vi "QueryMarker.vi"(8 "error in (no error)":errorcluster, 11 "Keysight44xx in":refnum<class "Keysight44xx.lvclass">) -> (0 "error out":errorcluster, 1 "MarkerPosition":dbl, 2 "MarkerAmplitude":dbl, 3 "Keysight44xx out":refnum<class "Keysight44xx.lvclass">)   [LabVIEW 2018, in "SpecAnPlugins.lvlib" / "Keysight44xx.lvclass"]
uses:
  Keysight44xx.lvclass
  C:/Users/ico/Documents/Projects/NistPluggableModules/SpecAn/SpecAnPlugins/SpecAnBaseClass/SpecAnBase.lvclass
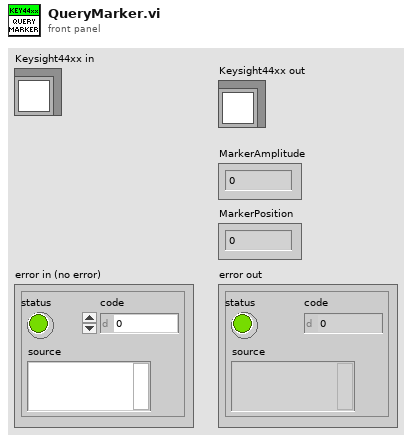
[diagram p1: front panel]
types:
  T1 = typedef "SpecAnPlugins.lvlib/SpecAnBase.lvclass/Acquisition.ctl" = cluster{"Handle":string, "Connected":bool, "Enabled":bool, "SweepModeContinuous":bool, "NumberOfSweeps":i32, "DetectorTypeAuto":bool, "DetectorType":i32, "VerticalScale":i32, "MaximumTime(seconds)":dbl}
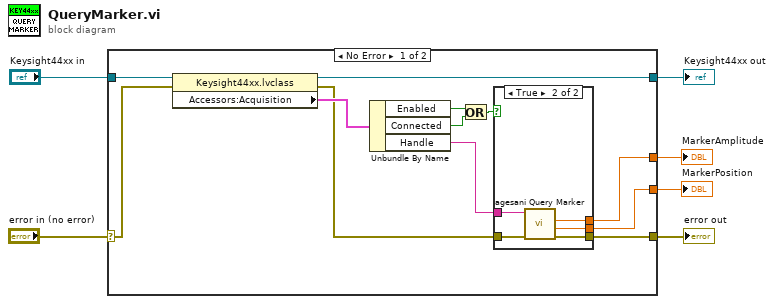
[diagram p0: block diagram]
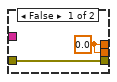
[diagram p2: hidden frame]
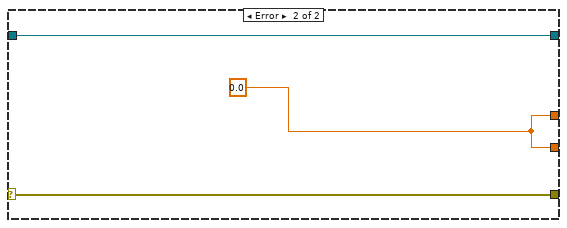
[diagram p3: hidden frame]
diagram:
  n1 = case shown="No Error" "error in (no error)" {
    selector: "error in (no error)" -> [w17 w27]
    tunnel: "Keysight44xx in" -> [w18 w28]
    tunnel: [w16 w28] -> w4
    tunnel: [w13 w27] -> w3
    tunnel: [w11 w26] -> w2
    tunnel: [w12 w26] -> w1
    frame No Error {
      n2 = property class="Keysight44xx.lvclass"(reference=w18, error in=w17) -> (reference out=w16:refnum<class "Keysight44xx.lvclass">, error out=w10:errorcluster, "Accessors:Acquisition"=w15:T1)
      n3 = Unbundle By Name(w15) -> ("Enabled"=w9:bool, "Connected"=w8:bool, "Handle"=w14:string)
      n4 = Or(x=w9, y=w8) -> (x .or. y?=w7:bool)
      n5 = case shown="True" w7 {
        tunnel: w14 -> [_ w25]
        tunnel: [w19 w24] -> w13
        tunnel: [w20 w23] -> w12
        tunnel: [w20 w22] -> w11
        tunnel: w10 -> [w19 w21]
        frame False {
          w20 = 0.0 ("marker amplitude")
        }
        frame True {
          n6 = call <instrlib>:"agesani Query Marker.vi"("error in (no error)"=w21, "instrument handle"=w25) -> ("error out"=w24:errorcluster, "marker position"=w23:dbl, "marker amplitude"=w22:dbl)  [unwired: 6 in, 1 out]
        }
      }
    }
    frame Error {
      w26 = 0.0 ("MarkerAmplitude")
    }
  }
  "error out" <- w3
  "Keysight44xx out" <- w4
  "MarkerAmplitude" <- w2
  "MarkerPosition" <- w1
